vi "Clear Log Before RSSI.vi"(6 "2.45 GHz Wake-Up Power":i8(ring)=6 items=["-29"=-29, "-4"=-4, "-2"=-2, "0"=0, "2"=2, "4"=4, "6"=6, "8"=8, "10"=10, "12"=12, "14"=14, "16"=16, "18"=18, "20"=20, "22"=22, "24"=24, "26"=26, "27"=27], 8 "error in":errorcluster, 9 "Attenuation dB (0)":dbl, 10 "400 MHz MICS Power Setting":u8=22 format="%.0x", 11 "VISA Resource Name":refnum<visa-resource-name>) -> (0 "error out":errorcluster, 3 "dup VISA Resource Name":refnum<visa-resource-name>)   [LabVIEW 2010]
uses:
  Typedef Command List.ctl
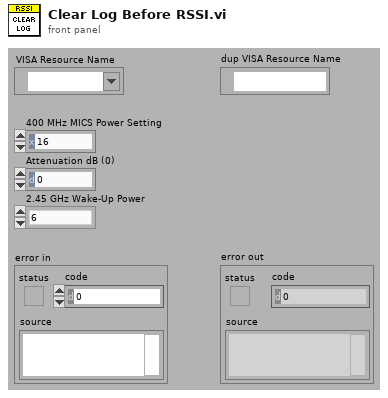
[diagram p1: front panel]
types:
  T1 = typedef "Typedef Command List.ctl" = enum16{"Get xPG Status", "xPG Stimulation", "Select Program", "Increment Program Amplitude", "Decrement Program Amplitude", "Get PoP Constants", "Get PPC Constants", "Get Program Names", "Set Pulse Amplitude", "Increment Pulse Amplitude", "Decrement Pulse Amplitude", "Get Pulse Widths", "Set Pulse Widths", "Increment Pulse Width", "Decrement Pulse Width", "Get Program Frequency", "Set Program Frequency", "Increment Program Frequency", "Decrement Program Frequency", "Inject Event", "Charging Control", "Get xPG Identity", "Set xPG Identity", "Restore Program Defaults", "Get Program Definition", "Set Program Definition", "Get Program Constants", "Set Program Constants", "Get Configurable Device Parameters", "Set Configurable Device Parameters", "Get Pulse Constants", "Set Pulse Constants", "Get Lead Limits", "Set Lead Limits", "Get Channel Calibrations", "Set Channel Calibrations", "<reserved 2>", "<reserved 3>", "<reserved 4>", "<reserved 5>", "<reserved 6>", "<reserved 7>", "Get Stim Asic HV Calibrations", "Set Stim Asic HV Calibrations", "<reserved 8>", "<reserved 9>", "Get CP Data", "Set CP Data", "Clear Log", "Read Log", "Append Log", "Get Patient Program Runtime", "Set Patient Program Runtime", "Impedance Measurement", "Enter Storage Mode", "Echo Short", "Echo Long", "Get General Calibration", "Set General Calibration", "Get Trim List", "Set Trim List", "Get Counter", "Set Counter", "Get Test Stimulation", "Set Test Stimulation", "Get Titration Stimulation", "Set Titration Stimulation", "Get Ramp Time", "Set Ramp Time", "Get VBAT", "Set Software Description Block", "Get Software Description Block", "Write Memory", "Read Memory", "Reset xPG", "Erase Flash Block", "Write Vectors", "Read Vectors", "Diagnostic Data", "Set Background Impedance", "Get Background Impedence ", "Set Test Waveform", "Calibrate Channel", "Get Log Range", "Reserved 0x55", "Reserved 0x56", "MICS Options", "Pair PPC", "Pair POP", "Stop Bootloader", "Tune MICS", "MICS Diagnostics", "Undefined"}
  T2 = cluster{"Command":T1, "Function":enum16{"Open Session", "Close Session", "Downlink Only", "Uplink Only", "Transceive (DN -> UP)"}, "MICS_ID":u32, "EXID":u32, "Use Local":bool, "Transceive Delay mS":dbl, "CP_DATA IN":u8[], "Parameters":string}
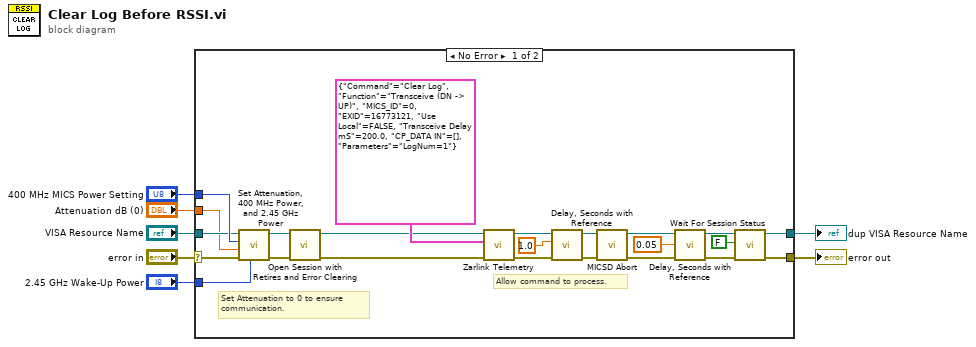
[diagram p0: block diagram]
diagram:
  n1 = case shown="No Error" "error in" {
    selector: "error in" -> [w13 w31]
    tunnel: "400 MHz MICS Power Setting" -> [w27 _]
    tunnel: "VISA Resource Name" -> [w26 w30]
    tunnel: "Attenuation dB (0)" -> [w22 _]
    tunnel: [w20 w30] -> w4
    tunnel: [w19 w31] -> w3
    tunnel: "2.45 GHz Wake-Up Power" -> [w18 _]
    frame No Error {
      # "Allow command to process."
      # "Set Attenuation to 0 to ensure\ncommunication."
      n2 = call "Set Attenuation, 400 MHz Power, and 2.45 GHz Power.vi"("2.45 GHz Wake-Up Power (6)"=w18, "error in"=w13, "Attenuation dB (0)"=w22, "400 MHz MICS Power Setting (0x16)"=w27, "VISA Resource Name"=w26) -> ("error out"=w16:errorcluster, "dup VISA Resource Name"=w17:refnum<visa-resource-name>)  [unwired: 5 in]
      n3 = call "Open Session with Retires and Error Clearing.vi"("error in"=w16, "VISA Resource Name"=w17) -> ("error out"=w15:errorcluster, "dup VISA Resource Name"=w14:refnum<visa-resource-name>)  [unwired: 6 in, 2 out]
      n4 = call "Zarlink Telemetry.vi"("error in (no error)"=w15, "Input"=T2 {"Command"=enum."Clear Log", "Function"=enum."Transceive (DN -> UP)", "MICS_ID"=0, "EXID"=16773121, "Use Local"=FALSE, "Transceive Delay mS"=200.0, "CP_DATA IN"=[], "Parameters"="LogNum=1"}, "MICS Dongle Address"=w14) -> ("error out"=w24:errorcluster)  [unwired: 6 in, 2 out]
      n5 = call "Delay, Seconds with Reference.vi"("error in"=w24, "delay"=dbl[unit] 1.0, "VISA resource"=w14) -> ("error out"=w29:errorcluster, "VISA resource dup"=w28:refnum<visa-resource-name>)  [unwired: 3 in, 1 out]
      n6 = call "MICSD Abort.vi"("error in (no error)"=w29, "VISA Resource Name"=w28) -> ("error out"=w10:errorcluster, "dup VISA Resource Name"=w12:refnum<visa-resource-name>)  [unwired: 8 in]
      n7 = call "Delay, Seconds with Reference.vi"("error in"=w10, "delay"=dbl[unit] 0.05, "VISA resource"=w12) -> ("error out"=w9:errorcluster, "VISA resource dup"=w11:refnum<visa-resource-name>)  [unwired: 3 in, 1 out]
      n8 = call "Wait For Session Status.vi"("error in (no error)"=w9, "IN_SESSION State (T)"=FALSE, "VISA Resource Name"=w11) -> ("error out"=w19:errorcluster, "dup VISA Resource Name"=w20:refnum<visa-resource-name>)  [unwired: 5 in, 2 out]
    }
    frame Error {
    }
  }
  "error out" <- w3
  "dup VISA Resource Name" <- w4
